vi "visualise.vi"(8 "error in (no error)":errorcluster, 11 "dataTA in":refnum<class "dataTA.lvclass">) -> (0 "error out":errorcluster, 3 "dataTA out":refnum<class "dataTA.lvclass">)   [LabVIEW 2019, in "dataTA.lvlib" / "dataTA.lvclass"]
uses:
  dataTA.lvclass
  dataTA.lvclass/dataTA.ctl
panel:
  in  "ampl":cluster{dbl, dbl}(slide)={-0.2917505030181087, 7321.931589537222} scale=-2000.0..16384.0
  in  "diff":dbl(slide)=26.080281690140847 scale=0.0..499.45051158551445
  out "XY Graph":T1(graph)
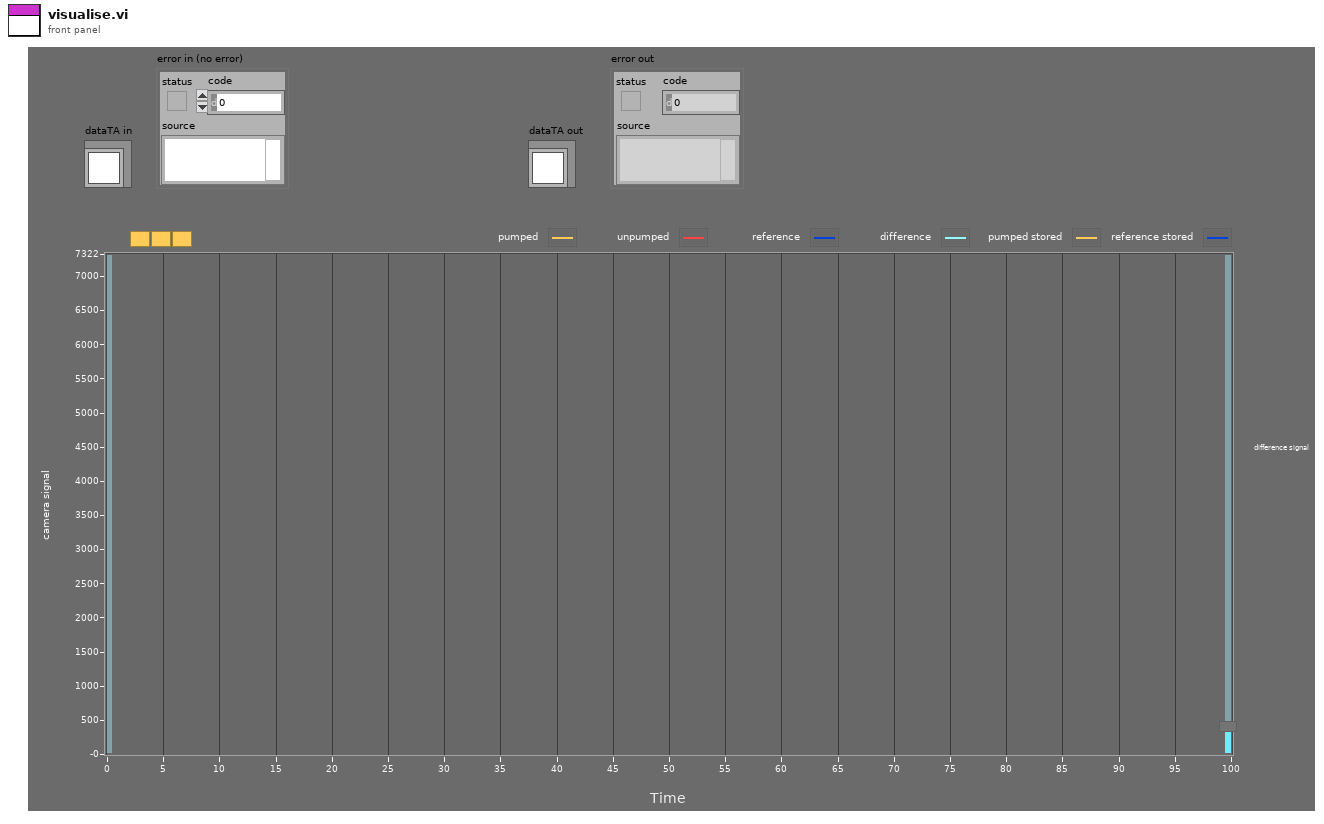
[diagram p1: front panel]
types:
  T1 = cluster{"wavelength":dbl[], "TA spectrum":dbl[]}[]
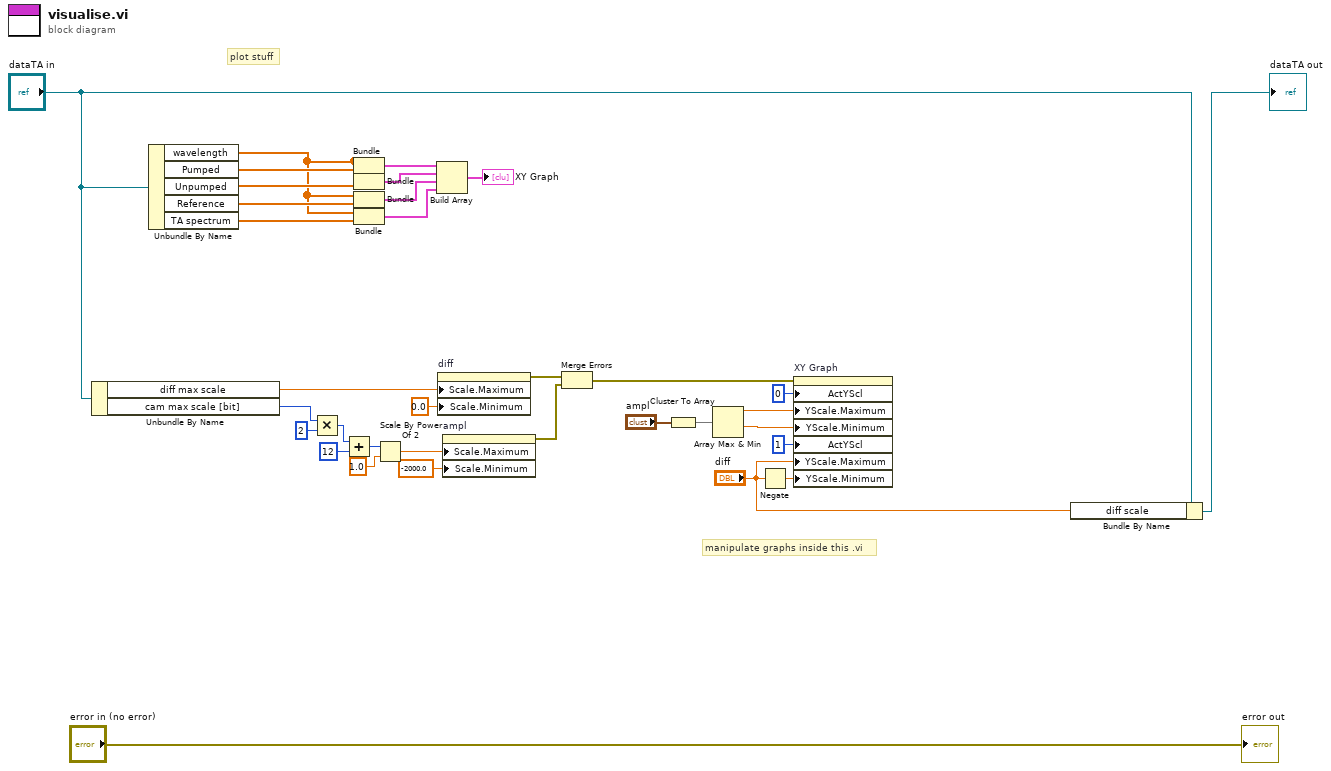
[diagram p0: block diagram]
diagram:
  # "plot stuff"
  # "manipulate graphs inside this .vi"
  n1 = Unbundle By Name("dataTA in") -> ("diff max scale"=w16:dbl, "cam max scale [bit]"=w15:u16)
  n2 = Unbundle By Name("dataTA in") -> ("wavelength"=w28:dbl[], "Pumped"=w33:dbl[], "Unpumped"=w30:dbl[], "Reference"=w29:dbl[], "TA spectrum"=w17:dbl[])
  n3 = Multiply(x=w15, y=2) -> (x*y=w13:i32)
  n4 = Add(x=w13, y=12) -> (x+y=w11:i32)
  n5 = Bundle("wavelength"=w28, "Pumped"=w33) -> (w32:cluster{"wavelength":dbl[], "Pumped":dbl[]})  [unwired: 1 in]
  n6 = Bundle("wavelength"=w28, "Unpumped"=w30) -> (w27:cluster{"wavelength":dbl[], "Unpumped":dbl[]})  [unwired: 1 in]
  n7 = Bundle("wavelength"=w28, "Reference"=w29) -> (w26:cluster{"wavelength":dbl[], "Reference":dbl[]})  [unwired: 1 in]
  n8 = Bundle("wavelength"=w28, "TA spectrum"=w17) -> (w25:cluster{"wavelength":dbl[], "TA spectrum":dbl[]})  [unwired: 1 in]
  n9 = Scale By Power Of 2(n=w11, x=1.0) -> (x*2^n=w10:dbl)
  n10 = Build Array(w32, w27, w26, w25) -> (→"XY Graph":T1)
  n11 = property on="diff" class="Slide (strict)"("Scale.Maximum"=w16, "Scale.Minimum"=0.0 ("Scale.Range:Minimum")) -> (error out=w7:errorcluster)  [unwired: 2 in, 1 out]
  n12 = property on="ampl" class="Slide (strict)"("Scale.Maximum"=w10, "Scale.Minimum"=-2000.0 ("Scale.Range:Minimum")) -> (error out=w6:errorcluster)  [unwired: 2 in, 1 out]
  n13 = Merge Errors(w7, w6) -> (w5:errorcluster)
  n14 = Cluster To Array(cluster="ampl") -> (array=w20:dbl[])
  n15 = Array Max & Min(array=w20) -> (max value=w19:dbl, min value=w18:dbl)  [unwired: 2 out]
  n16 = Negate(x="diff") -> (-x=w22:dbl)
  n17 = property on="XY Graph" class="XYGraph (strict)"(error in=w5, "ActYScl"=0 ("Active Y Scale"), "YScale.Maximum"=w19, "YScale.Minimum"=w18, "ActYScl"=1 ("Active Y Scale"), "YScale.Maximum"="diff", "YScale.Minimum"=w22) -> ()  [unwired: 1 in, 2 out]
  n18 = Bundle By Name(cluster="dataTA in", "diff scale"="diff") -> (→"dataTA out":refnum<class "dataTA.lvclass">)
  "error out" <- "error in (no error)"
